vi "Find Tests - Error Input - Returns No Test Cases.vi"() -> ()   [LabVIEW 2017, in "LVUnit Test Discoverer.Tests.lvlib"]
uses:
  LVUnit Test Discoverer.Tests.lvlib
  LVUnit Test Discoverer/LVUnit Test Discoverer.lvclass
  Assertion/Assertion.lvlib
  Test Case/Test Case.lvclass
panel:
  out "error out":errorcluster
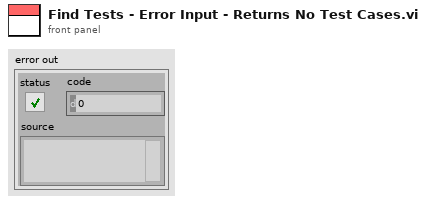
[diagram p1: front panel]
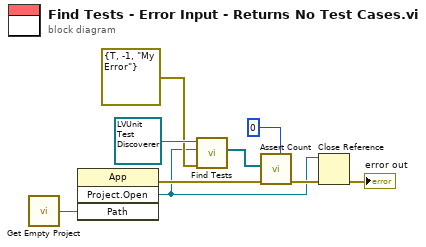
[diagram p0: block diagram]
diagram:
  n1 = call "Get Empty Project.vi"() -> ("Project File"=w8:path)  [unwired: 2 in]
  n2 = invoke class="App" method="Project.Open"("Path"=w8) -> (error out=w6:errorcluster, "Project:Open"=w1:refnum<vi>)  [unwired: 3 in, 2 out]
  n3 = call-dynamic "Find Tests.vi"("error in (no error)"=errorcluster {"status"=TRUE, "code"=-1, "source"="My Error"} ("error constant"), "Project Refnum"=w1, "LVUnit Test Discoverer in"=refnum<class "LVUnit Test Discoverer.lvclass"> refnum ("LVUnit Test Discoverer")) -> ("Test Cases"=w4:refnum<class "Test Case.lvclass">[])  [unwired: 6 in, 2 out]
  n4 = call "Assert Count.vi"("Expected"=0, "error in (no error)"=w6, "Haystack"=w4) -> ("error out"=w5:errorcluster)  [unwired: 8 in]
  n5 = Close Reference(reference=w1, error in (no error)=w5) -> (error out=→"error out":errorcluster)
